vi "Unwrap2DwithMask.vi"   [LabVIEW 2015]
types:
  T1 = typedef "NI_Matrix.lvlib/RealMatrix.ctl" = dbl[][]
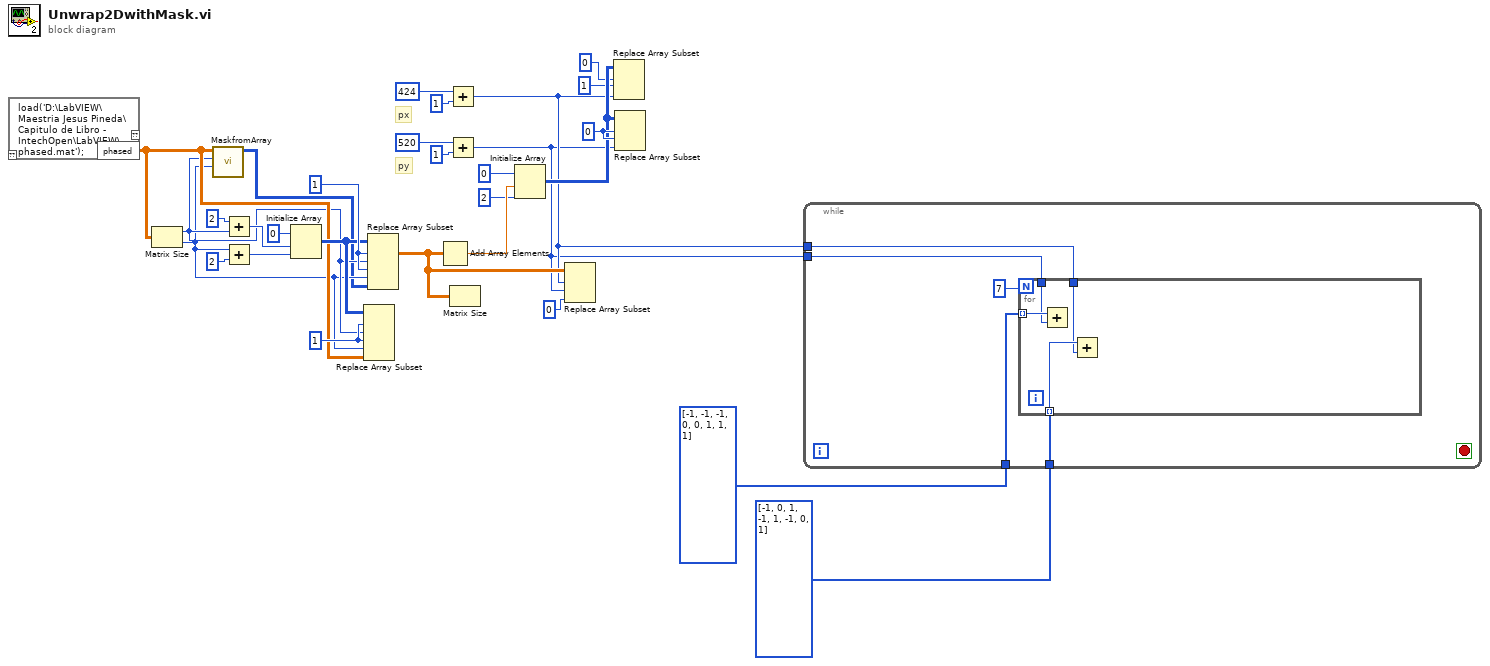
[diagram p0: block diagram]
diagram:
  w10 = 0
  w18 = 1
  w21 = 1
  # "px"
  # "py"
  n1 = script code="load('D:\\LabVIEW\\Maestria Jesus Pineda\\Capitulo de Libro - IntechOpen\\LabVIEW\\phased.mat');"() -> ("phased"=w17:dbl[][])  [unwired: 1 in, 1 out]
  n2 = Matrix Size(0:w17) -> (1:w16:i32, 2:w15:i32)
  n3 = call "MaskfromArray.vi"("cols"=w15, "rows"=w16, "Array"=w17) -> ("Image Pixels (U8)"=w14:u8[][])  [unwired: 8 in]
  n4 = Add(x=2, y=w16) -> (x+y=w22:i32)
  n5 = Add(x=w15, y=2) -> (x+y=w20:i32)
  n6 = Initialize Array(0, w22, w20) -> (w19:i32[][])
  n7 = Replace Array Subset(array=w19, new element=w17, index (dim 0)=w18, index (dim 1)=w16, index (dim 2)=w18, index (dim 3)=w15) -> ()  [unwired: 1 out]
  n8 = Replace Array Subset(array=w19, new element=w14, index (dim 0)=w21, index (dim 1)=w16, index (dim 2)=w21, index (dim 3)=w15) -> (w6:T1)
  n9 = Add Array Elements(numeric array=w6) -> (sum=w13:dbl)
  n10 = Add(x=424, y=1) -> (x+y=w4:i32)
  n11 = Add(x=520, y=1) -> (x+y=w3:i32)
  n12 = Matrix Size(0:w6) -> ()  [unwired: 2 out]
  n13 = Initialize Array(0, w13, 2) -> (w9:i32[][])
  n14 = Replace Array Subset(array=w6, new element=0, index (row)=w4, index (col)=w3) -> ()  [unwired: 1 out]
  n15 = Replace Array Subset(array=w9, new element=w4, index (row)=0, index (col)=1) -> ()  [unwired: 1 out]
  n16 = Replace Array Subset(array=w9, new element=w3, index (row)=w10, index (col)=w10) -> ()  [unwired: 1 out]
  n17 = while {
    tunnel: w4 -> [w30]
    tunnel: w3 -> [w32]
    tunnel: i32[] [-1, -1, -1, 0, 0, 1, 1, 1] -> [w33]
    tunnel: i32[] [-1, 0, 1, -1, 1, -1, 0, 1] -> [w31]
    stop <- _ stop-if-true
    n18 = for {
      N: 7 -> [_]
      tunnel: w33 -> [w38] mode=indexing
      tunnel: w32 -> [w37]
      tunnel: w31 -> [w36] mode=indexing
      tunnel: w30 -> [w35]
      n19 = Add(x=w38, y=w37) -> ()  [unwired: 1 out]
      n20 = Add(x=w36, y=w35) -> ()  [unwired: 1 out]
    }
  }
